vi "InitMap.vi"(10 "key values":string[](array[string]), 11 "key names":string[](array[string])) -> (3 "Map":map{i32, u8[]}(c390))   [LabVIEW 2023, in "LP_CRC.lvlib"]
uses:
  LP_CRC.lvlib
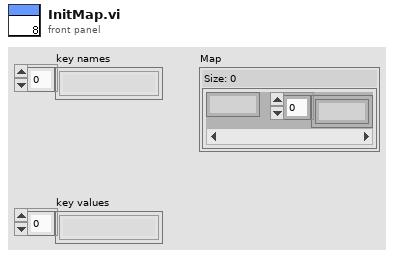
[diagram p1: front panel]
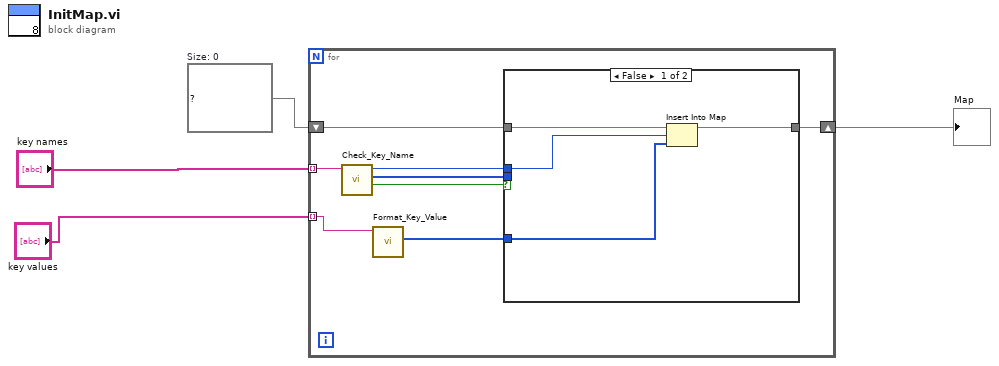
[diagram p0: block diagram]
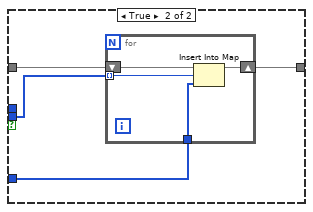
[diagram p2: hidden frame]
diagram:
  w2 = map{i32, u8[]} {}  # Size: 0
  n1 = for {
    tunnel: "key names" -> [w12] mode=indexing
    shift-right: [w11] -> w4
    shift-left: w2 -> [w7]
    tunnel: "key values" -> [w6] mode=indexing
    n2 = call "Check_Key_Name.vi"("String"=w12) -> ("multi?"=w10:bool, "IDs"=w8:u32[], "ID"=w9:u32)  [unwired: 8 in]
    n3 = call "Format_Key_Value.vi"("value"=w6) -> ("key value"=w5:u32[])  [unwired: 9 in, 1 out]
    n4 = case shown="False" w10 {
      tunnel: [w16 w19] -> w11
      tunnel: w9 -> [w14 _]
      tunnel: w8 -> [_ w18]
      tunnel: w7 -> [w15 w20]
      tunnel: w5 -> [w13 w17]
      frame False {
        n5 = Insert Into Map(map in=w15, key=w14, value=w13) -> (map out=w16:map{i32, u8[]})  [unwired: 2 out]
      }
      frame True {
        n6 = for {
          shift-right: [w23] -> w19
          shift-left: w20 -> [w24]
          tunnel: w18 -> [w22] mode=indexing
          tunnel: w17 -> [w21]
          n7 = Insert Into Map(map in=w24, key=w22, value=w21) -> (map out=w23:map{i32, u8[]})  [unwired: 2 out]
        }
      }
    }
  }
  "Map" <- w4
